vi "Y_Stage.vi"() -> ()   [LabVIEW 2013]
panel:
  out "Current X Position":sgl
  in  "Serial 3":i32=90848556
  in  "MG17Motor 3":refnum<k7>(container)
  in  "Y-Coordinate":dbl
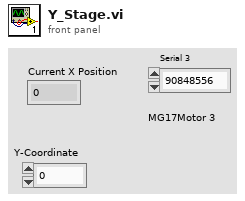
[diagram p1: front panel]
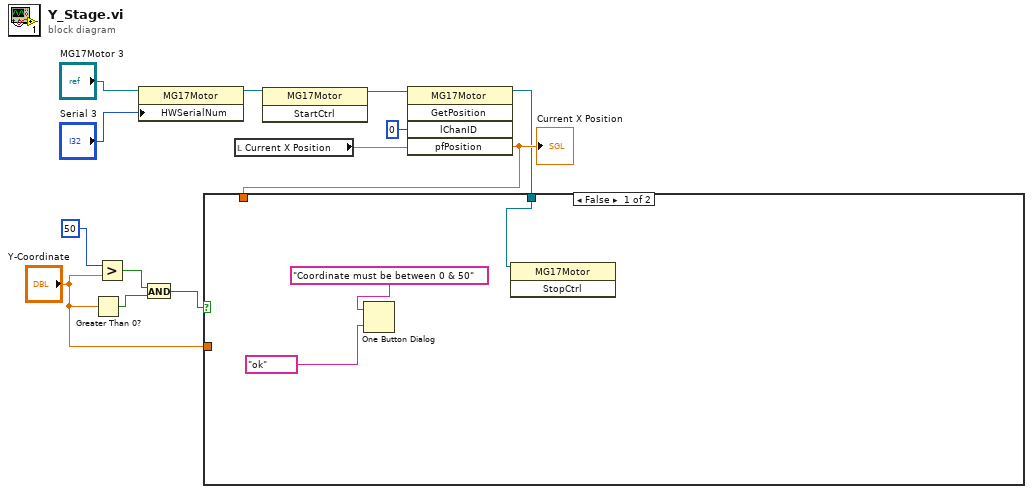
[diagram p0: block diagram]
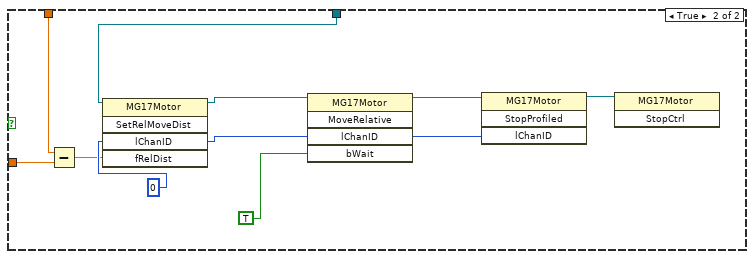
[diagram p2: hidden frame]
diagram:
  n1 = Greater Than 0?(x="Y-Coordinate") -> (x > 0?=w7:bool)
  n2 = Greater?(x=50, y="Y-Coordinate") -> (0:w6:bool)
  n3 = property class="MG17Motor"(reference="MG17Motor 3", "HWSerialNum"="Serial 3") -> (reference out=w11:refnum<k7>)  [unwired: 1 in, 1 out]
  n4 = And(x=w6, y=w7) -> (x .and. y?=w2:bool)
  n5 = local read "Current X Position"() -> (w8:sgl)
  n6 = invoke class="MG17Motor" method="StartCtrl"(reference=w11) -> (reference out=w9:refnum<k7>)  [unwired: 2 in, 2 out]
  n7 = invoke class="MG17Motor" method="GetPosition"(reference=w9, "lChanID"=0, "pfPosition"=w8) -> (reference out=w1:refnum<k7>, "pfPosition"=w3:sgl)  [unwired: 2 in, 3 out]
  "Current X Position" <- w3
  n8 = case shown="False" w2 {
    tunnel: "Y-Coordinate" -> [_ w20]
    tunnel: w3 -> [_ w19]
    tunnel: w1 -> [w16 w17]
    frame False {
      n9 = One Button Dialog(message="Coordinate must be between 0 & 50", button name ("OK")="ok") -> ()  [unwired: 1 out]
      n10 = invoke class="MG17Motor" method="StopCtrl"(reference=w16) -> ()  [unwired: 2 in, 3 out]
    }
    frame True {
      n11 = Subtract(x=w19, y=w20) -> (x-y=w18:dbl)
      n12 = invoke class="MG17Motor" method="SetRelMoveDist"(reference=w17, "lChanID"=0, "fRelDist"=w18) -> (reference out=w23:refnum<k7>, "lChanID"=w24:i32)  [unwired: 2 in, 3 out]
      n13 = invoke class="MG17Motor" method="MoveRelative"(reference=w23, "lChanID"=w24, "bWait"=TRUE) -> (reference out=w25:refnum<k7>, "lChanID"=w26:i32)  [unwired: 2 in, 3 out]
      n14 = invoke class="MG17Motor" method="StopProfiled"(reference=w25, "lChanID"=w26) -> (reference out=w27:refnum<k7>)  [unwired: 2 in, 3 out]
      n15 = invoke class="MG17Motor" method="StopCtrl"(reference=w27) -> ()  [unwired: 2 in, 3 out]
    }
  }
